vi "录音机实验.vi"() -> ()   [LabVIEW 2011]
panel:
  out "Recording Time（S）":u16 max=64
  in  "保存":bool
  out "数值":i32
  in  "暂停":bool
  out "Create_Success?":bool
  in  "录音":bool
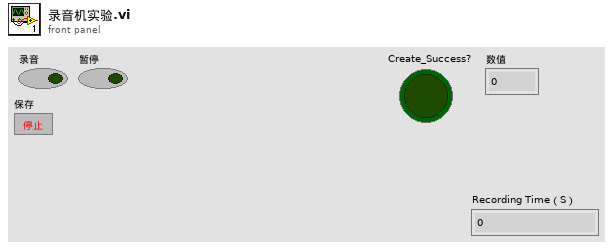
[diagram p1: front panel]
types:
  T1 = enum8{"P0", "P1", "P2", "P3", "P4", "P5", "P6", "P7", "P8", "P9", "P10", "P11", "P12", "P13", "P14", "P15"}
  T2 = enum8{"Port_A", "Port_B", "Port_C", "Port_D", "Port_E", "Port_F", "Port_G", "Port_H", "Port_I"}
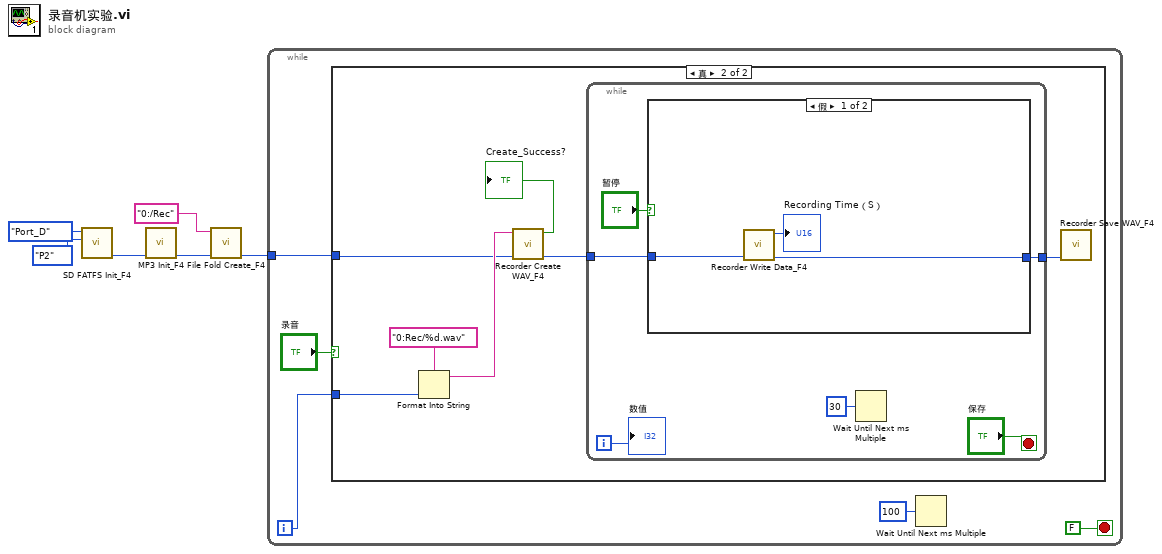
[diagram p0: block diagram]
diagram:
  n1 = call <vilib>:"SD FATFS Init_F4.vi"("SD_CS_pin"=T1."P2", "SD_CS_PortX"=T2."Port_D") -> ("err_out"=w1:u8)  [unwired: 8 in, 1 out]
  n2 = call <vilib>:"MP3 Init_F4.vi"("err_in"=w1) -> ("err_out"=w2:u8)  [unwired: 10 in]
  n3 = call <vilib>:"File Fold Create_F4.vi"("err_in"=w2, "Fold Path"="0:/Rec") -> ("err_out"=w3:u8)  [unwired: 8 in, 1 out]
  n4 = while {
    tunnel: w3 -> [w10]
    i -> [w9]
    stop <- FALSE stop-if-true
    n5 = case shown="真" "录音" {
      tunnel: w10 -> [_ w15]
      tunnel: w9 -> [_ w18]
      frame False {
      }
      frame True {
        n6 = Format Into String(format string="0:Rec/%d.wav" ("格式字符串"), w18) -> (resulting string=w16:string)  [unwired: 2 in, 1 out]
        n7 = call <vilib>:"Recorder Create WAV_F4.vi"("err_in"=w15, "Recorder WAV Path"=w16) -> ("err_out"=w13:u8, "Create_Success?"=→"Create_Success?":bool)  [unwired: 8 in]
        n8 = while {
          tunnel: w13 -> [w23]
          tunnel: [w22] -> w12
          i -> [w21]
          stop <- "保存" stop-if-true
          n9 = case shown="假" "暂停" {
            tunnel: w23 -> [w26 _]
            tunnel: [w25 _] -> w22
            frame False {
              n10 = call <vilib>:"Recorder Write Data_F4.vi"("err_in"=w26) -> ("err_out"=w25:u8, "Recording Time（S）"=→"Recording Time（S）":u16)  [unwired: 9 in]
            }
            frame True {
            }
          }
          n11 = Wait Until Next ms Multiple(millisecond multiple=u32 30 ("毫秒倍数")) -> ()  [unwired: 1 out]
          "数值" <- w21
        }
        n12 = call <vilib>:"Recorder Save WAV_F4.vi"("err_in"=w12) -> ()  [unwired: 10 in, 1 out]
      }
    }
    n13 = Wait Until Next ms Multiple(millisecond multiple=u32 100 ("毫秒倍数")) -> ()  [unwired: 1 out]
  }
